vi "Random 2D Array.vi"() -> ()   [LabVIEW 2012]
uses:
  demo dll.dll
panel:
  out "波形图":dbl[][](graph)
  in  "停止":bool
  in  "max":dbl=1.0
  in  "min":dbl
  in  "col":i32=4
  in  "row":i32=3
  out "Array2D":dbl[][](array[numeric])=[[0.3918495053190256, 0.87385885559352, 0.050258167765520945, 0.33648502938600977], [1.102149171397729, 1.1119314435829442, 1.2975484304319365, 1.7352063295002425], [2.3126051475434304, 2.6509011689452606, 2.6193012557482964, 2.5911250359206663]]
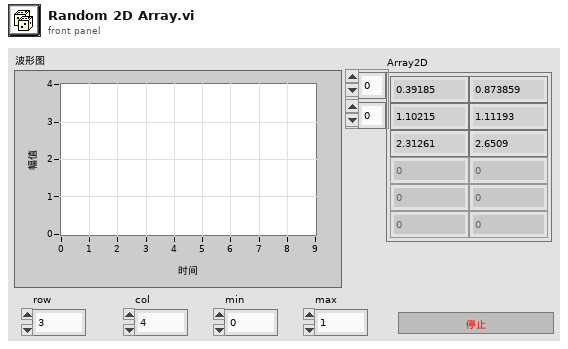
[diagram p1: front panel]
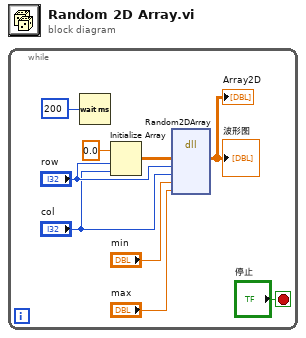
[diagram p0: block diagram]
diagram:
  n1 = while {
    stop <- "停止" stop-if-true
    n2 = Wait (ms)(milliseconds to wait=u32 200 ("等待时间（毫秒）")) -> ()  [unwired: 1 out]
    n3 = Initialize Array(0.0 ("元素"), "row", "col") -> (w9:dbl[][])
    n4 = dll-call lib="PTH1+abs EBOOK\t功能块DLLdemo dll.dll" fn="Random2DArray"("Array2D"=w9, "row"="row", "col"="col", "min"="min", "max"="max") -> ("Array2D"=→"Array2D" →"波形图":dbl[][])  [unwired: 8 in, 2 out]
  }
